vi "RS232.vi"() -> ()   [LabVIEW 2014]
uses:
  <vilib>/Instr/_visa.llb/VISA Configure Serial Port (Instr).vi
panel:
  out "连接的字符串":string
  in  "命令值":i32=592700
  out "错误输出 1":errorcluster caption="错误输出"
  in  "VISA resource name 1":refnum<visa-resource-name>="COM3" caption="VISA资源名称"
  in  "baud rate (9600) 1":u32=115200 caption="波特率(9600)"
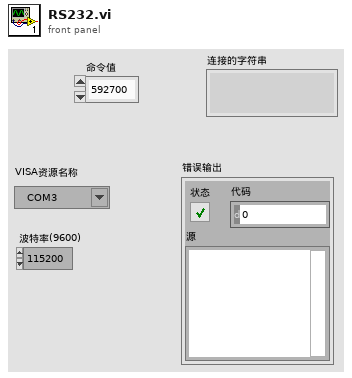
[diagram p1: front panel]
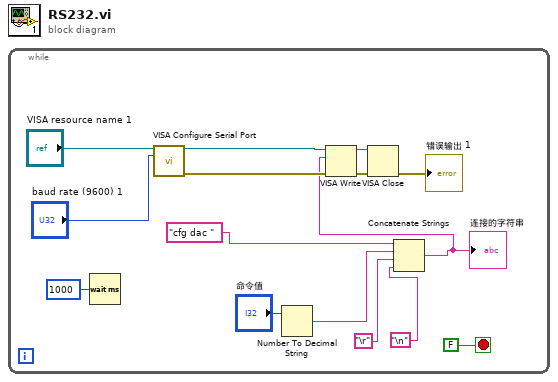
[diagram p0: block diagram]
diagram:
  n1 = while {
    stop <- FALSE stop-if-true
    n2 = Wait (ms)(milliseconds to wait=u32 1000 ("等待时间（毫秒）")) -> ()  [unwired: 1 out]
    n3 = call-poly "VISA Configure Serial Port"("VISA resource name"="VISA resource name 1", "baud rate (9600)"="baud rate (9600) 1") -> ("VISA resource name out"=w15:refnum<visa-resource-name>, "error out"=w12:errorcluster)  [unwired: 12 in]
    n4 = Number To Decimal String(number="命令值") -> (decimal integer string=w6:string)  [unwired: 1 in]
    n5 = Concatenate Strings("cfg dac " ("写入缓冲区"), w6, "\r", "\n") -> (w3:string)
    "连接的字符串" <- w3
    n6 = VISA Write(VISA resource name=w15, write buffer=w3, error in (no error)=w12) -> (VISA resource name out=w13:refnum<visa-resource-name>, error out=w11:errorcluster)  [unwired: 1 out]
    n7 = VISA Close(VISA resource name=w13, error in (no error)=w11) -> (error out=→"错误输出 1":errorcluster)
  }
